vi "AVS_Temp-Monitor.vi"   [LabVIEW 2016]
uses:
  data/Data_Display_global.vi
  Instrument_Setup_v2.vi
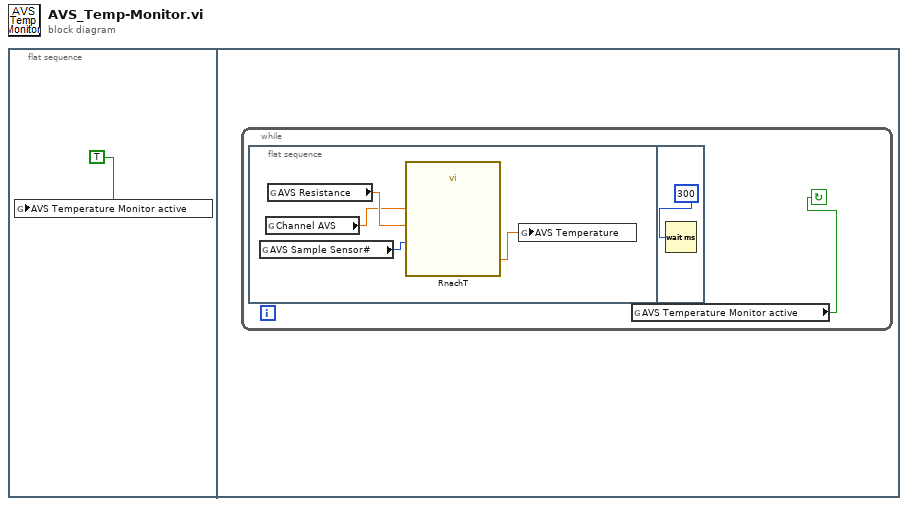
[diagram p0: block diagram]
diagram:
  n1 = flat-sequence {
    frame #0 {
      n2 = global write "Data_Display_global.vi" "AVS Temperature Monitor active"(TRUE) -> ()
    }
    frame #1 {
      n3 = while {
        stop <- w2 continue-if-true
        n4 = flat-sequence {
          frame #0 {
            n5 = global read "Instrument_Setup_v2.vi" "AVS Sample Sensor#"() -> (w5:u16)
            n6 = global read "Instrument_Setup_v2.vi" "Channel AVS"() -> (w3:dbl)
            n7 = global read "Data_Display_global.vi" "AVS Resistance"() -> (w6:dbl)
            n8 = call "RnachT.vi"("AVS Channel"=w3, "R"=w6, "Sensor Cal#"=w5) -> ("T (K)"=w4:dbl)
            n9 = global write "Data_Display_global.vi" "AVS Temperature"(w4) -> ()
          }
          frame #1 {
            n10 = Wait (ms)(milliseconds to wait=300) -> ()  [unwired: 1 out]
          }
        }
        n11 = global read "Data_Display_global.vi" "AVS Temperature Monitor active"() -> (w2:bool)
      }
    }
  }
